vi "Not Boolean Array (16).vi"() -> ()   [LabVIEW 2010]
doc: "This VI performs not operation on Boolean Array of Size 16"
panel:
  out "Not X":bool[](array[boolean])
  in  "X":bool[](array[boolean])=[FALSE, FALSE, FALSE, FALSE, FALSE, FALSE, FALSE, TRUE, FALSE, FALSE, FALSE, FALSE, FALSE, FALSE, FALSE, FALSE]
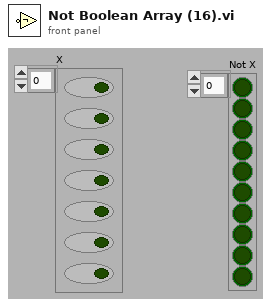
[diagram p1: front panel]
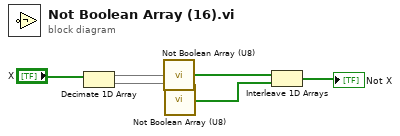
[diagram p0: block diagram]
diagram:
  n1 = Decimate 1D Array("X") -> (w5:bool[], w4:bool[])
  n2 = call "Not Boolean Array (U8).vi"("X"=w5) -> ("Not X"=w3:bool[])  [unwired: 4 in]
  n3 = call "Not Boolean Array (U8).vi"("X"=w4) -> ("Not X"=w2:bool[])  [unwired: 4 in]
  n4 = Interleave 1D Arrays(w3, w2) -> (→"Not X":bool[])
